vi "LinMot Test.vi"() -> ()   [LabVIEW 2018]
uses:
  LabVIEW_ProducerConsumer/COM_ComModule.lvlibp/LT_Config.ctl
  LabVIEW_ProducerConsumer/COM_ComModule.lvlibp
panel:
  in  "Rueckwaerts":T1={"Pos [mm]"=10.0, "Speed [m/s]"=0.1, "Acc [m/s^2]"=1.0, "Dec [m/s^2]"=1.0}
  in  "Vorwärts":T1={"Pos [mm]"=10.0, "Speed [m/s]"=0.1, "Acc [m/s^2]"=1.0, "Dec [m/s^2]"=1.0}
  in  "LT Cfg in":T2
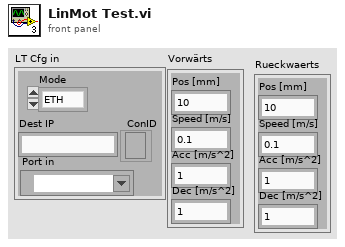
[diagram p1: front panel]
types:
  T1 = cluster{"Pos [mm]":dbl, "Speed [m/s]":dbl, "Acc [m/s^2]":dbl, "Dec [m/s^2]":dbl}
  T2 = typedef "COM_ComModule.lvlibp/LT_Config.ctl" = cluster{"Mode":enum16{"ETH", "RS"}, "Dest IP":string, "ConID":refnum<k16>, "Port in":refnum<visa-resource-name>}
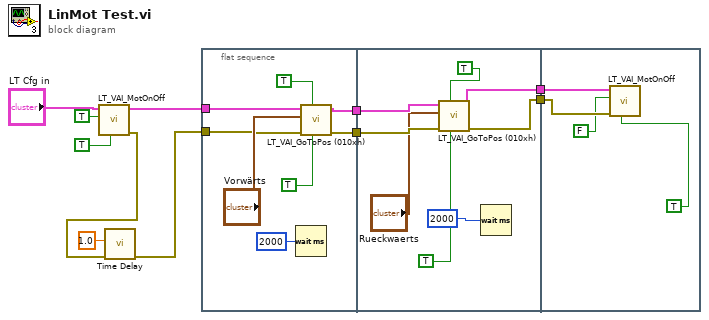
[diagram p0: block diagram]
diagram:
  n1 = call "LT_VAI_MotOnOff.vi"("open/close"=TRUE, "Mot on/off"=TRUE, "LT Cfg in"="LT Cfg in") -> ("error out"=w3:errorcluster, "LT Cfg out"=w10:T2)  [unwired: 7 in]
  n2 = call "Time Delay"("error in (no error)"=w3, "Delay Time (s)"=1.0) -> ("error out"=w2:errorcluster)  [unwired: 9 in]
  n3 = flat-sequence {
    tunnel: w10 -> [w17]
    tunnel: w2 -> [w16]
    tunnel: [w14] -> w7
    tunnel: [w13] -> w6
    tunnel: w7 -> [w24]
    tunnel: w6 -> [w25]
    tunnel: [w23] -> w5
    tunnel: [w22] -> w4
    tunnel: w5 -> [w30]
    tunnel: w4 -> [w28]
    frame #0 {
      n4 = Wait (ms)(milliseconds to wait=u32 2000) -> ()  [unwired: 1 out]
      n5 = call "LT_VAI_GoToPos (010xh).vi"("open/close"=TRUE, "Wait for Motion"=TRUE, "error in"=w16, "VAI Par"="Vorwärts", "LT Cfg in"=w17) -> ("error out"=w13:errorcluster, "LT Cfg out"=w14:T2)  [unwired: 5 in]
    }
    frame #1 {
      n6 = call "LT_VAI_GoToPos (010xh).vi"("open/close"=TRUE, "Wait for Motion"=TRUE, "error in"=w25, "VAI Par"="Rueckwaerts", "LT Cfg in"=w24) -> ("error out"=w23:errorcluster, "LT Cfg out"=w22:T2)  [unwired: 5 in]
      n7 = Wait (ms)(milliseconds to wait=u32 2000) -> ()  [unwired: 1 out]
    }
    frame #2 {
      n8 = call "LT_VAI_MotOnOff.vi"("open/close"=TRUE, "error in"=w30, "Mot on/off"=FALSE, "LT Cfg in"=w28) -> ()  [unwired: 6 in, 2 out]
    }
  }
